vi "DangerEnemy.vi"(10 "IA Input":T1={"our_robots"=[], "enemy_robots"=[], "balls"=[], "geometry"={"line_width"=0, "field_length"=0, "field_width"=0, "boundary_width"=0, "referee_width"=0, "goal_width"=0, "goal_depth"=0, "goal_wall_width"=0, "center_circle_radius"=0, "defense_radius"=0, "defense_stretch"=0, "free_kick_from_defense_dist"=0, "penalty_spot_from_field_line_dist"=0, "penalty_line_from_spot_dist"=0}, "IA Judge"={"stage"="", "command"="", "our_goalie_id"=0.0, "enemy_goalie_id"=0.0, "command enum"=enum."Halt", "Time"=enum."Azul"}, "Received Timestamp"=timestamp(0 s since 1904-01-01), "Events"={"Touch"=FALSE, "Ball out"=FALSE, "id touch"=0.0, "Ball out of \nVision"=FALSE, "Ball inside \nGoalie area"=FALSE, "Robot not responding"=FALSE, "Robots responding status"=[1.0, 1.0, 1.0, 1.0, 1.0, 1.0], "Enemy Ball \nPossession"=FALSE, "Pass State"=FALSE, "id end of pass"=0.0, "Kick"=FALSE, "Id ini Possession"=0.0, "Ball Possesion"=FALSE, "Id Possesion"=0.0}}) -> (1 "Pos do inimigo\nperigoso":dbl[](array[numeric]), 2 "id do inimigo\nmais perigoso":u32)   [LabVIEW 2017]
uses:
  Core/AI Input.ctl
  Core/AI Robot.ctl
  Functions Enum.ctl
  AttackerStates.ctl
  Core/AI Ball.ctl
  Core/Field Size.ctl
  Core/AI Judge.ctl
  Command Enum.ctl
  Util/Events/Events.ctl
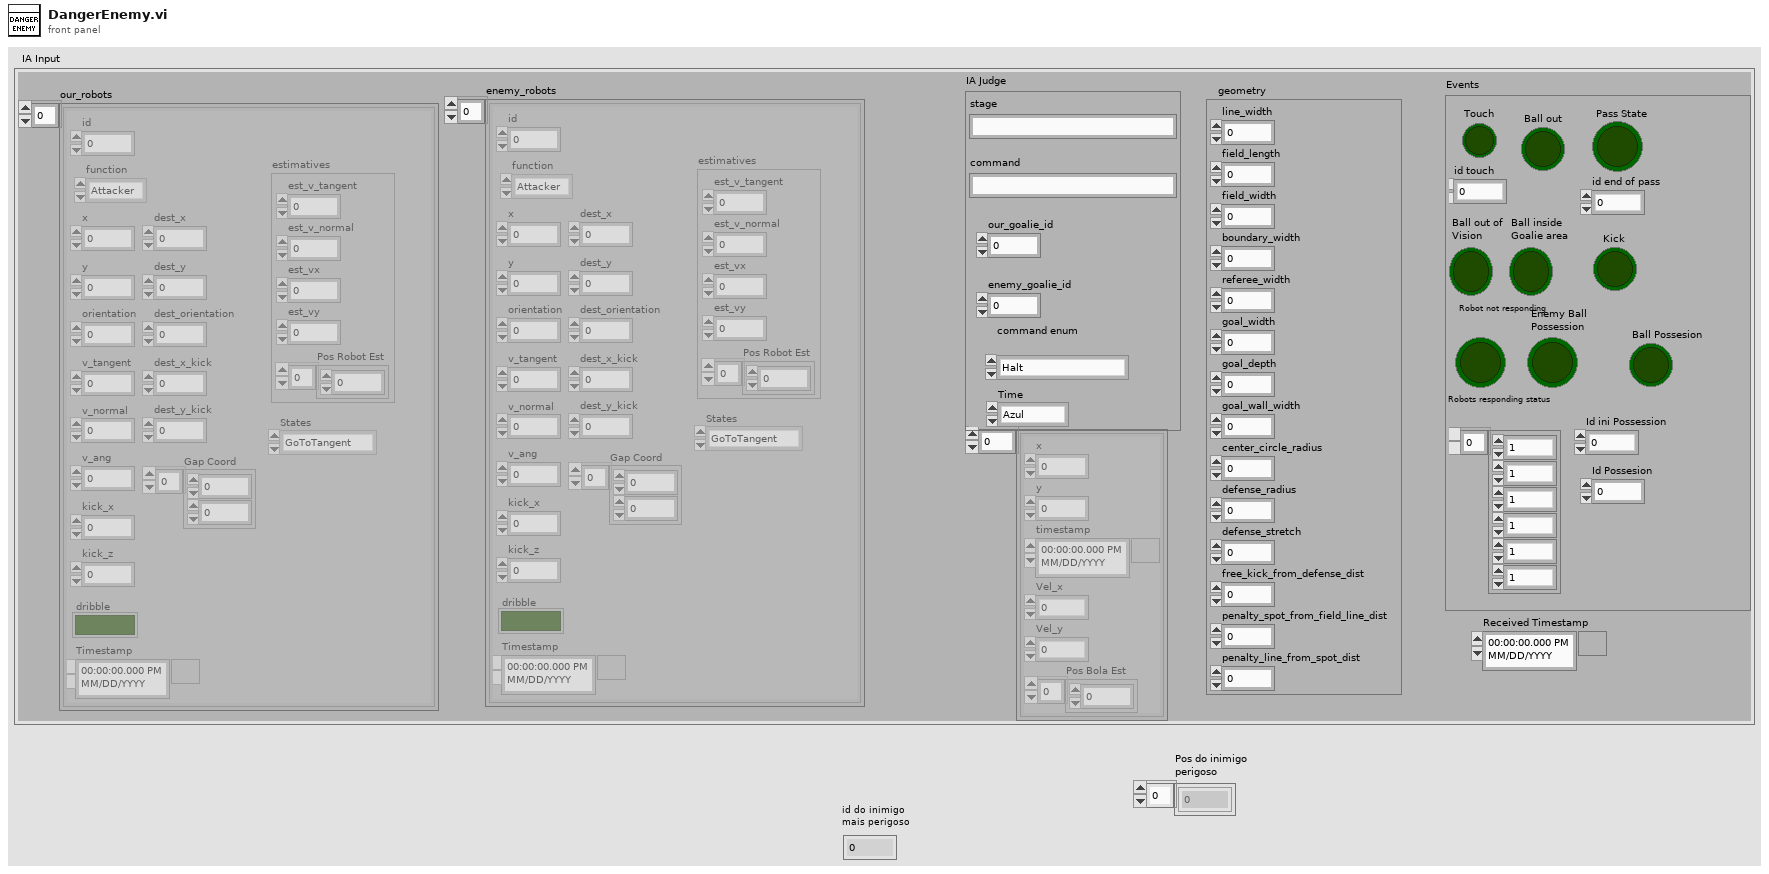
[diagram p1: front panel]
types:
  T1 = typedef "AI Input.ctl" = cluster{"our_robots":T2[], "enemy_robots":T2[], "balls":T5[], "geometry":T6, "IA Judge":T7, "Received Timestamp":timestamp, "Events":T9}
  T2 = typedef "AI Robot.ctl" = cluster{"id":u32, "function":T3, "x":dbl, "y":dbl, "orientation":dbl, "v_tangent":dbl, "v_normal":dbl, "v_ang":dbl, "kick_x":dbl, "kick_z":dbl, "dribble":bool, "Timestamp":timestamp, "dest_x":dbl, "dest_y":dbl, "dest_orientation":dbl, "estimatives":cluster{"est_v_tangent":dbl, "est_v_normal":dbl, "est_vx":dbl, "est_vy":dbl, "Pos Robot Est":dbl[]}, "dest_x_kick":dbl, "dest_y_kick":dbl, "Gap Coord":dbl[], "States":T4}
  T3 = typedef "Functions Enum.ctl" = enum16{"Attacker", "Goalie", "Defender", "Striker", "Goto 0", "Dummy", "Kicker", "ZigZag"}
  T4 = typedef "AttackerStates.ctl" = enum16{"Pass", "GoToTangent", "BallGetting", "GoToKick", ""}
  T5 = typedef "AI Ball.ctl" = cluster{"x":dbl, "y":dbl, "timestamp":timestamp, "Vel_x":dbl, "Vel_y":dbl, "Pos Bola Est":dbl[]}
  T6 = typedef "Field Size.ctl" = cluster{"line_width":u32, "field_length":u32, "field_width":u32, "boundary_width":u32, "referee_width":u32, "goal_width":u32, "goal_depth":u32, "goal_wall_width":u32, "center_circle_radius":u32, "defense_radius":u32, "defense_stretch":u32, "free_kick_from_defense_dist":u32, "penalty_spot_from_field_line_dist":u32, "penalty_line_from_spot_dist":u32}
  T7 = typedef "AI Judge.ctl" = cluster{"stage":string, "command":string, "our_goalie_id":dbl, "enemy_goalie_id":dbl, "command enum":T8, "Time":enum16{"Azul", "Amarelo"}}
  T8 = typedef "Command Enum.ctl" = enum16{"Halt", "Stop", "Force Start", "PKA Normal Start", "Prepare Kickoff Ally", "PKE Normal Start", "Prepare Kickoff Enemy", "Prepare Penalty Ally", "PPA Normal Start", "Prepare Penalty Enemy", "PPE Normal Start", "Direct Free Enemy", "Direct Free Ally", "Indirect Free Enemy", "Indirect Free Ally", "Timeout Enemy", "Timeout Ally", "Goal Enemy", "Goal Ally", "Ball Placement Enemy", "Ball Placement Ally", "Normal Half Time", "Extra Time Break", "Extra Half Time", "None", "Post Game"}
  T9 = typedef "Events.ctl" = cluster{"Touch":bool, "Ball out":bool, "id touch":dbl, "Ball out of \nVision":bool, "Ball inside \nGoalie area":bool, "Robot not responding":bool, "Robots responding status":dbl[], "Enemy Ball \nPossession":bool, "Pass State":bool, "id end of pass":dbl, "Kick":bool, "Id ini Possession":dbl, "Ball Possesion":bool, "Id Possesion":dbl}
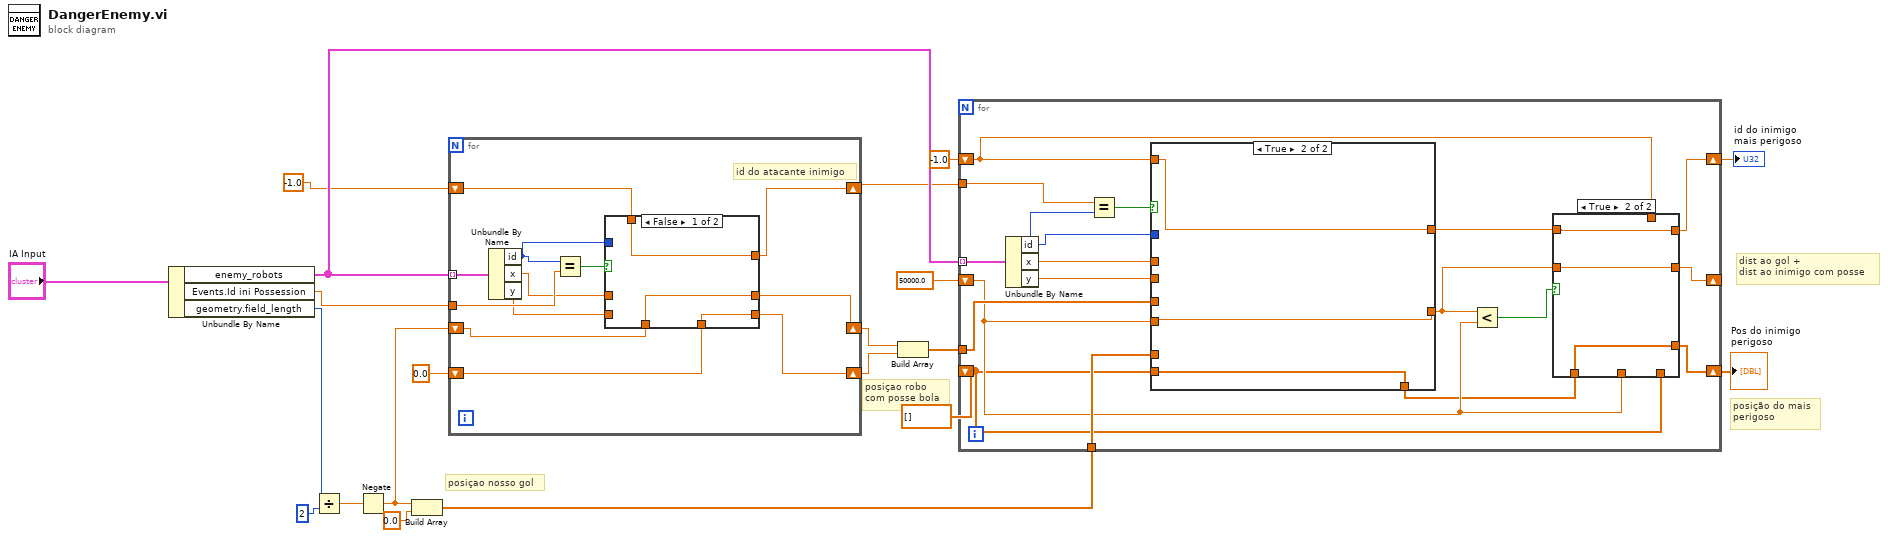
[diagram p0: block diagram]
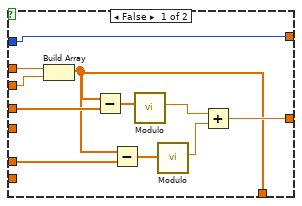
[diagram p3: hidden frame]
diagram:
  # "dist ao gol +\ndist ao inimigo com posse"
  # "posição do mais\nperigoso"
  # "posiçao nosso gol"
  # "posiçao robo\ncom posse bola"
  n1 = Unbundle By Name("IA Input") -> ("enemy_robots"=w18:T2[], "Events.Id ini Possession"=w19:dbl, "geometry.field_length"=w13:u32)
  n2 = Divide(x=w13, y=u32 2) -> (x/y=w11:dbl)
  n3 = Negate(x=w11) -> (-x=w1:dbl)
  n4 = Build Array(w1, 0.0 ("element")) -> (w9:dbl[])
  n5 = for {
    tunnel: w18 -> [w32] mode=indexing
    tunnel: w19 -> [w31]
    shift-right: [w26] -> w17
    shift-left: -1.0 ("id") -> [w23]
    shift-right: [w25] -> w16
    shift-left: w1 -> [w22]
    shift-right: [w24] -> w15
    shift-left: 0.0 ("y") -> [w21]
    # "id do atacante inimigo"
    n6 = Unbundle By Name(w32) -> ("id"=w29:u32, "x"=w28:dbl, "y"=w27:dbl)
    n7 = Equal?(x=w29, y=w31) -> (x = y?=w30:bool)
    n8 = case shown="False" w30 {
      tunnel: w29 -> [_ w38]
      tunnel: w28 -> [_ w37]
      tunnel: w27 -> [_ w36]
      tunnel: [w35 w38] -> w26
      tunnel: [w34 w37] -> w25
      tunnel: [w33 w36] -> w24
      tunnel: w23 -> [w35 _]
      tunnel: w22 -> [w34 _]
      tunnel: w21 -> [w33 _]
      frame False {
      }
      frame True {
      }
    }
  }
  n9 = Build Array(w16, w15) -> (w14:dbl[])
  n10 = for {
    tunnel: w18 -> [w56] mode=indexing
    tunnel: w17 -> [w55]
    tunnel: w14 -> [w51]
    tunnel: w9 -> [w50]
    shift-right: [w47] -> _
    shift-left: 50000.0 -> [w46]
    shift-right: [w43] -> w7
    shift-left: -1.0 ("id") -> [w40]
    shift-right: [w41] -> w6
    shift-left: dbl[] [] -> [w39]
    n11 = Unbundle By Name(w56) -> ("id"=w45:u32, "x"=w53:dbl, "y"=w52:dbl)
    n12 = Equal?(x=w55, y=w45) -> (x = y?=w54:bool)
    n13 = case shown="True" w54 {
      tunnel: w53 -> [w73 _]
      tunnel: w52 -> [w72 _]
      tunnel: w51 -> [w71 _]
      tunnel: w50 -> [w69 _]
      tunnel: [w65 w76] -> w48
      tunnel: w46 -> [_ w76]
      tunnel: w45 -> [w64 _]
      tunnel: [w64 w75] -> w44
      tunnel: [w63 w74] -> w42
      tunnel: w40 -> [_ w75]
      tunnel: w39 -> [_ w74]
      frame False {
        n14 = Build Array(w73, w72) -> (w63:dbl[])
        n15 = Subtract(x=w63, y=w71) -> (x-y=w70:dbl[])
        n16 = Subtract(x=w63, y=w69) -> (x-y=w68:dbl[])
        n17 = call "Modulo.vi"("2D vector"=w70) -> ("Modulo"=w67:dbl)  [unwired: 10 in]
        n18 = call "Modulo.vi"("2D vector"=w68) -> ("Modulo"=w66:dbl)  [unwired: 10 in]
        n19 = Add(x=w67, y=w66) -> (x+y=w65:dbl)
      }
      frame True {
      }
    }
    n20 = Less?(x=w48, y=w46) -> (x < y?=w49:bool)
    n21 = case shown="True" w49 {
      tunnel: w48 -> [_ w62]
      tunnel: [w59 w62] -> w47
      tunnel: w46 -> [w59 _]
      tunnel: [w58 w61] -> w43
      tunnel: w44 -> [_ w61]
      tunnel: w40 -> [w58 _]
      tunnel: w42 -> [_ w60]
      tunnel: [w57 w60] -> w41
      tunnel: w39 -> [w57 _]
      frame False {
      }
      frame True {
      }
    }
  }
  "id do inimigo\nmais perigoso" <- w7
  "Pos do inimigo\nperigoso" <- w6
